vi "Write Relays.vi"(8 "error in (no error)":errorcluster, 10 "Relays":refnum<class "Relay.lvclass">[](array[class]), 11 "Switch Action Processor in":refnum<class "Switch Action Processor.lvclass">) -> (0 "error out":errorcluster, 3 "Switch Action Processor out":refnum<class "Switch Action Processor.lvclass">)   [LabVIEW 2015]
uses:
  Switch Action Processor.lvclass
  Relay/Relay.lvclass
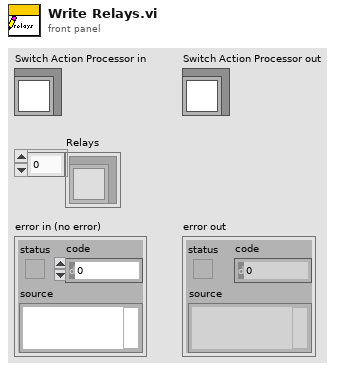
[diagram p1: front panel]
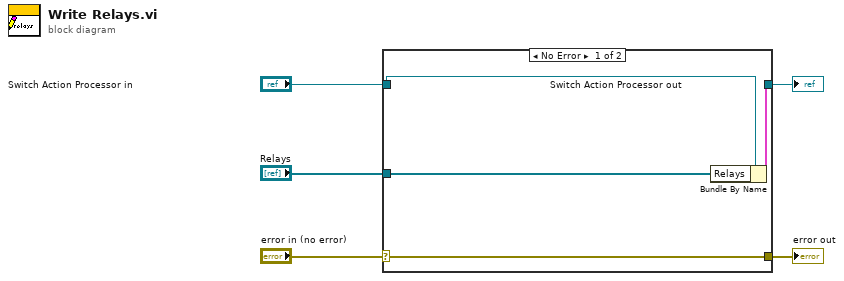
[diagram p0: block diagram]
diagram:
  n1 = case shown="No Error" "error in (no error)" {
    selector: "error in (no error)" -> [w9 w10]
    tunnel: [w9 w10] -> w4
    tunnel: [w7 w11] -> w2
    tunnel: "Switch Action Processor in" -> [w8 w11]
    tunnel: "Relays" -> [w6 _]
    frame No Error {
      n2 = Bundle By Name(cluster=w8, "Relays"=w6) -> (w7:cluster{})
    }
    frame Error {
    }
  }
  "error out" <- w4
  "Switch Action Processor out" <- w2
